vi "Do Core.vi"(8 "error in (no error)":errorcluster, 9 "Actor in":refnum<class "Actor.lvclass">, 11 "Reply Message":refnum<class "Read RandomNum Msg.lvclass">) -> (0 "error out":errorcluster, 1 "Actor out":refnum<class "Actor.lvclass">, 2 "Reply":variant)   [LabVIEW 2021, in "Generator.lvlib" / "Read RandomNum Msg.lvclass"]
doc: "(<B>Filename</B>: Actor Framework.lvlib:Reply Msg.lvclass:Do Core.vi)\n\nDefines what an actor does when it receives <B>Reply Message</B>. This method also defines the <B>Reply</B> that is returned to the actor that sent <B>Reply Message</B>.\n\nBy default, this method does nothing, and <B>Reply</B> is the ancestor Message class. A child class must override this method to define behavior and specify a child of the Message class to return in the <B>Reply</B> output."
uses:
  Read RandomNum Msg.lvclass
  <vilib>/ActorFramework/Actor/Actor.lvclass
  Generator/Generator.lvclass
  C:/Program Files (x86)/National Instruments/LabVIEW 2021/vi.lib/ActorFramework/Actor/Actor.lvclass
  Generator/Generator.lvclass/Generator.ctl
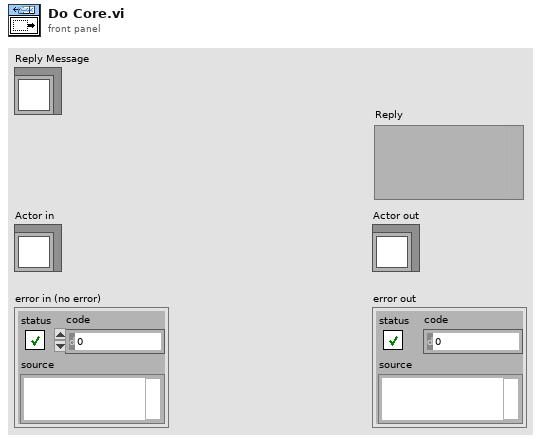
[diagram p1: front panel]
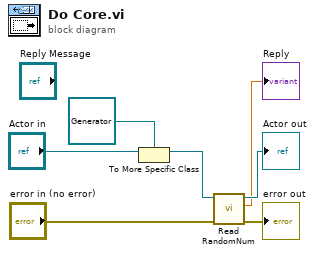
[diagram p0: block diagram]
diagram:
  n1 = To More Specific Class(target class=refnum<class "Generator.lvclass"> refnum ("Generator.lvlib:Generator.lvclass"), reference="Actor in") -> (specific class reference=w2:refnum<class "Generator.lvclass">)  [unwired: 1 in, 1 out]
  n2 = call "Read RandomNum.vi"("error in (no error)"="error in (no error)", "Generator in"=w2) -> ("error out"=→"error out":errorcluster, "RandomNum"=→"Reply":dbl, "Generator out"=→"Actor out":refnum<class "Generator.lvclass">)  [unwired: 7 in]
